vi "LIA Debugging FPGA.vi"() -> ()   [LabVIEW 2017]
uses:
  <instrlib>/_niInstr/Streaming/v1/Common/Stream State.ctl
  <instrlib>/_niInstr/Data Trigger/v1/Shared/Public/Edge Configuration FXP(+-,18,1).ctl
  <instrlib>/_niInstr/Data Trigger/v1/Shared/Public/Edge Configuration Trigger Slope.ctl
  LIA Decimator0 Enum.ctl
  LIA Decimator1 Enum.ctl
  Cascaded-SOS/FPGA/Controls/IIR_Coeffs.ctl
  <vilib>/Platform/TimedLoop/XDataNode/timing_clust.ctl
  <vilib>/Platform/TimedLoop/XDataNode/nitl_modes.ctl
  <vilib>/Platform/TimedLoop/XDataNode/wakeup.ctl
  <instrlib>/_niInstr/DSP/v1/Shared/Public/IQ Data.ctl
  <vilib>/rvi/Emulation/niFpgaSctlEmulationGetInTimedLoop.vi
  <vilib>/rvi/Emulation/niFpgaEmulationReportErrorSimple.vi
  <vilib>/rvi/Emulation/niFpgaGetClockAttributes.vi
  <vilib>/rvi/Emulation/niFpgaCriticalErrorInLSC.vi
  <instrlib>/_niInstr/DSP/v1/FPGA/Public/Sub VIs/Frequency Shift/Frequency Shift - 1 spc.vi
  <instrlib>/_niInstr/DSP/v1/FPGA/Public/Sub VIs/Fractional Decimator/Fractional Decimator - 1 spc - 2x oc.vi
  <instrlib>/_niInstr/DSP/v1/FPGA/Public/Sub VIs/Fractional Decimator/Fractional Decimator - 10 cps - 1x oc.vi
  <userlib>/_NI Noise Generation IP/FPGA/Public/Low Level/AWGN FXP23x2.vi
  <instrlib>/_niInstr/DSP/v1/FPGA/Public/Sub VIs/Frequency Shift/Frequency Shift - 2 spc.vi
  <vilib>/rvi/eio/common/nirviEmuTemplateMethod_errors.vi
  <vilib>/Platform/TimedLoop/XDataNode/XDataNode.xnode
  <instrlib>/_niInstr/DSP/v1/Xnodes/Public/Frequency Shift/niInstr DSP v1 Frequency Shift FPGA.xnode
  <vilib>/rvi/FXPMathLib/FxpMul/XNode/nifxpmath_Multiplier.xnode
  <vilib>/rvi/FXPMathLib/FxpAdd/XNode/nifxpmath_Add.xnode
  <vilib>/eio/EIONode/EIONode.xnode
  <vilib>/Platform/TimedLoop/XDataNode/XDNodeRunTimeDep.lvlib
  <instrlib>/_niInstr/Basic Elements/v1/FPGA/niInstr Basic Elements v1 FPGA.lvlib
  <instrlib>/_niInstr/DSP/v1/Shared/niInstr DSP v1 Shared.lvlib
  <instrlib>/_niInstr/DSP/v1/FPGA/niInstr DSP v1 FPGA.lvlib
  Program Files (x86)/National Instruments/LabVIEW 2017/examples/Lock-In Amplifier/_NI PLL IP/FPGA/NI PLL IP FPGA.lvlib
  Program Files (x86)/National Instruments/LabVIEW 2017/examples/Lock-In Amplifier/lib/fpga/Lock-In Amplifier Example FPGA.lvlib
  <instrlib>/_niInstr/Streaming/v1/Common/niInstr Streaming v1 Common.lvlib
  <userlib>/_NI Noise Generation IP/FPGA/NI Noise Generation IP FPGA v2.lvlib
  <vilib>/rvi/FXPMathLib/sim/FxpSim.dll
  <instrlib>/_niInstr/Data Trigger/v1/Shared/niInstr Data Trigger v1 Shared.lvlib
panel:
  in  "lock-in.iir enable0 0":bool
  in  "lock-in.iir enable1 0":bool
  in  "lock-in.iir config1 0":T1={"b0"=0.015777587890625, "b1"=-0.030517578125, "-a1"=1.9578399658203125, "-a2"=-0.9589080810546875}
  in  "lock-in.iir decimation1 0":fxp<+,4,4> format="%#_3g"
  in  "lock-in.iir decimation0 0":fxp<+,4,4> format="%#_3g"
  in  "lock-in.iir config0 0":T1={"b0"=0.015777587890625, "b1"=-0.030517578125, "-a1"=1.9578399658203125, "-a2"=-0.9589080810546875}
  in  "lock-in.decimator1 0":T2
  in  "lock-in.fir1 fs 0":fxp<+,48,1>
  in  "nco.enable 0":bool=TRUE
  in  "nco.reset 0":bool
  in  "nco.frequency 0":fxp<+/-,48,0>
  in  "lock-in.fir0 fs 0":fxp<+,48,1>
  in  "lock-in.decimator0 0":T3
  in  "dpll.reset 1":bool
  in  "dpll.enable 1":bool
  in  "dpll.q 1":fxp<+/-,48,0>
  in  "dpll.m 1":i8
  in  "dpll.config 1":T4
  out "dpll.vco output 1":fxp<+/-,48,0>
  in  "dpll.channel 1":i32
  in  "dpll.channel 0":i32
  out "dpll.vco output 0":fxp<+/-,48,0>
  in  "dpll.config 0":T4
  in  "dpll.m 0":i8
  in  "dpll.q 0":fxp<+/-,48,0>
  in  "dpll.enable 0":bool
  in  "dpll.reset 0":bool
  in  "lock-in.enable 3":bool
  in  "lock-in.enable 2":bool
  in  "lock-in.enable 1":bool
  in  "lock-in.carrier 3":fxp<+/-,48,0>
  in  "lock-in.carrier 2":fxp<+/-,48,0>
  in  "lock-in.enable 0":bool
  in  "lock-in.channel select 3":i32
  in  "lock-in.carrier select 3":i32
  in  "lock-in.cic config valid 3":bool
  in  "lock-in.cic config 3":cluster{"factor":fxp<+,16,16>, "shift":i16}
  in  "lock-in.reset 3":bool
  out "stream.state 3":T6 caption="stream.state 0"
  out "stream.samples transferred 3":u64 caption="stream.samples transferred 0"
  out "stream.metadata 3":u64 caption="stream.metadata 0"
  in  "stream.num samples 3":u64 caption="stream.num samples 0"
  in  "stream.request state 3":T6 caption="stream.request state 0"
  in  "lock-in.channel select 2":i32
  in  "lock-in.carrier select 2":i32
  in  "lock-in.cic config valid 2":bool
  in  "lock-in.cic config 2":cluster{"factor":fxp<+,16,16>, "shift":i16}
  in  "lock-in.reset 2":bool
  out "stream.state 2":T6 caption="stream.state 0"
  out "stream.samples transferred 2":u64 caption="stream.samples transferred 0"
  out "stream.metadata 2":u64 caption="stream.metadata 0"
  in  "stream.num samples 2":u64 caption="stream.num samples 0"
  in  "stream.request state 2":T6 caption="stream.request state 0"
  out "pll.vco output 0":fxp<+/-,48,0>
  out "pll.vco output 1":fxp<+/-,48,0>
  out "stream.metadata 4":u64 caption="stream.metadata 0"
  out "stream.samples transferred 4":u64 caption="stream.samples transferred 0"
  out "stream.state 4":T6 caption="stream.state 0"
  in  "stream.request state 4":T6 caption="stream.request state 0"
  in  "stream.num samples 4":u64 caption="stream.num samples 0"
  in  "preview.channel select":i32
  in  "ao.reset 3":bool
  in  "ao.carrier 2":fxp<+/-,48,0>=0.010000000000001563
  in  "ao.level 2":fxp<+/-,18,1>
  in  "ao.reset 2":bool
  in  "ao.carrier 1":fxp<+/-,48,0>=0.010000000000001563
  in  "ao.level 1":fxp<+/-,18,1>
  in  "ao.reset 1":bool
  in  "ao.reset 0":bool
  in  "ao.carrier 0":fxp<+/-,48,0>=0.010000000000001563
  in  "ao.level 0":fxp<+/-,18,1>
  in  "lock-in.channel select 1":i32
  in  "lock-in.channel select 0":i32
  in  "stream.request state 1":T6 caption="stream.request state 0"
  in  "stream.num samples 1":u64 caption="stream.num samples 0"
  out "stream.metadata 1":u64 caption="stream.metadata 0"
  out "stream.samples transferred 1":u64 caption="stream.samples transferred 0"
  out "stream.state 1":T6 caption="stream.state 0"
  in  "lock-in.reset 1":bool
  in  "lock-in.cic config 1":cluster{"factor":fxp<+,16,16>, "shift":i16}
  in  "lock-in.cic config valid 1":bool
  in  "lock-in.carrier select 1":i32
  in  "lock-in.carrier select 0":i32
  in  "lock-in.cic config valid 0":bool
  in  "lock-in.cic config 0":cluster{"factor":fxp<+,16,16>, "shift":i16}
  in  "lock-in.reset 0":bool
  in  "lock-in.carrier 1":fxp<+/-,48,0>
  in  "lock-in.carrier 0":fxp<+/-,48,0>
  in  "ao.level 3":fxp<+/-,18,1>
  in  "pll.channel 1":i32
  in  "pll.reset 1":bool
  in  "pll.enable 1":bool
  in  "pll.config 1":T7={"quiescent frequency"=0.10000000000000142, "compensation"=0.0, "psd gain"=-18, "loop filter"={"order"=4, "cutoff"=6}}
  in  "pll.channel 0":i32
  in  "ao.noise gain 3":fxp<+,18,1>=0.01000213623046875
  in  "ao.carrier 3":fxp<+/-,48,0>=0.010000000000001563
  in  "ao.noise seeds 3":fxp<+,23,23>[](array[numeric])=[1.0, 12323.0]
  in  "pll.reset 0":bool
  in  "pll.enable 0":bool
  in  "stream.request state 0":T6
  in  "stream.num samples 0":u64
  out "stream.metadata 0":u64
  out "stream.samples transferred 0":u64
  out "stream.state 0":T6
  in  "pll.config 0":T7={"quiescent frequency"=0.10000000000000142, "compensation"=0.0, "psd gain"=-18, "loop filter"={"order"=4, "cutoff"=6}}
  out "IO Module\\InitDone":bool
  out "IO Module\\User Error":u32
  in  "IO Module\\User Command":u32
  in  "IO Module\\User Command Valid":bool
  out "IO Module\\User Command Ready":bool
  in  "IO Module\\User Command Arg 0":u32
  in  "IO Module\\User Command Arg 1":u32
  out "IO Module\\User Command Error":u16
  out "IO Module\\User Command Return":u32
  out "IO Module\\User Command Return Valid":bool
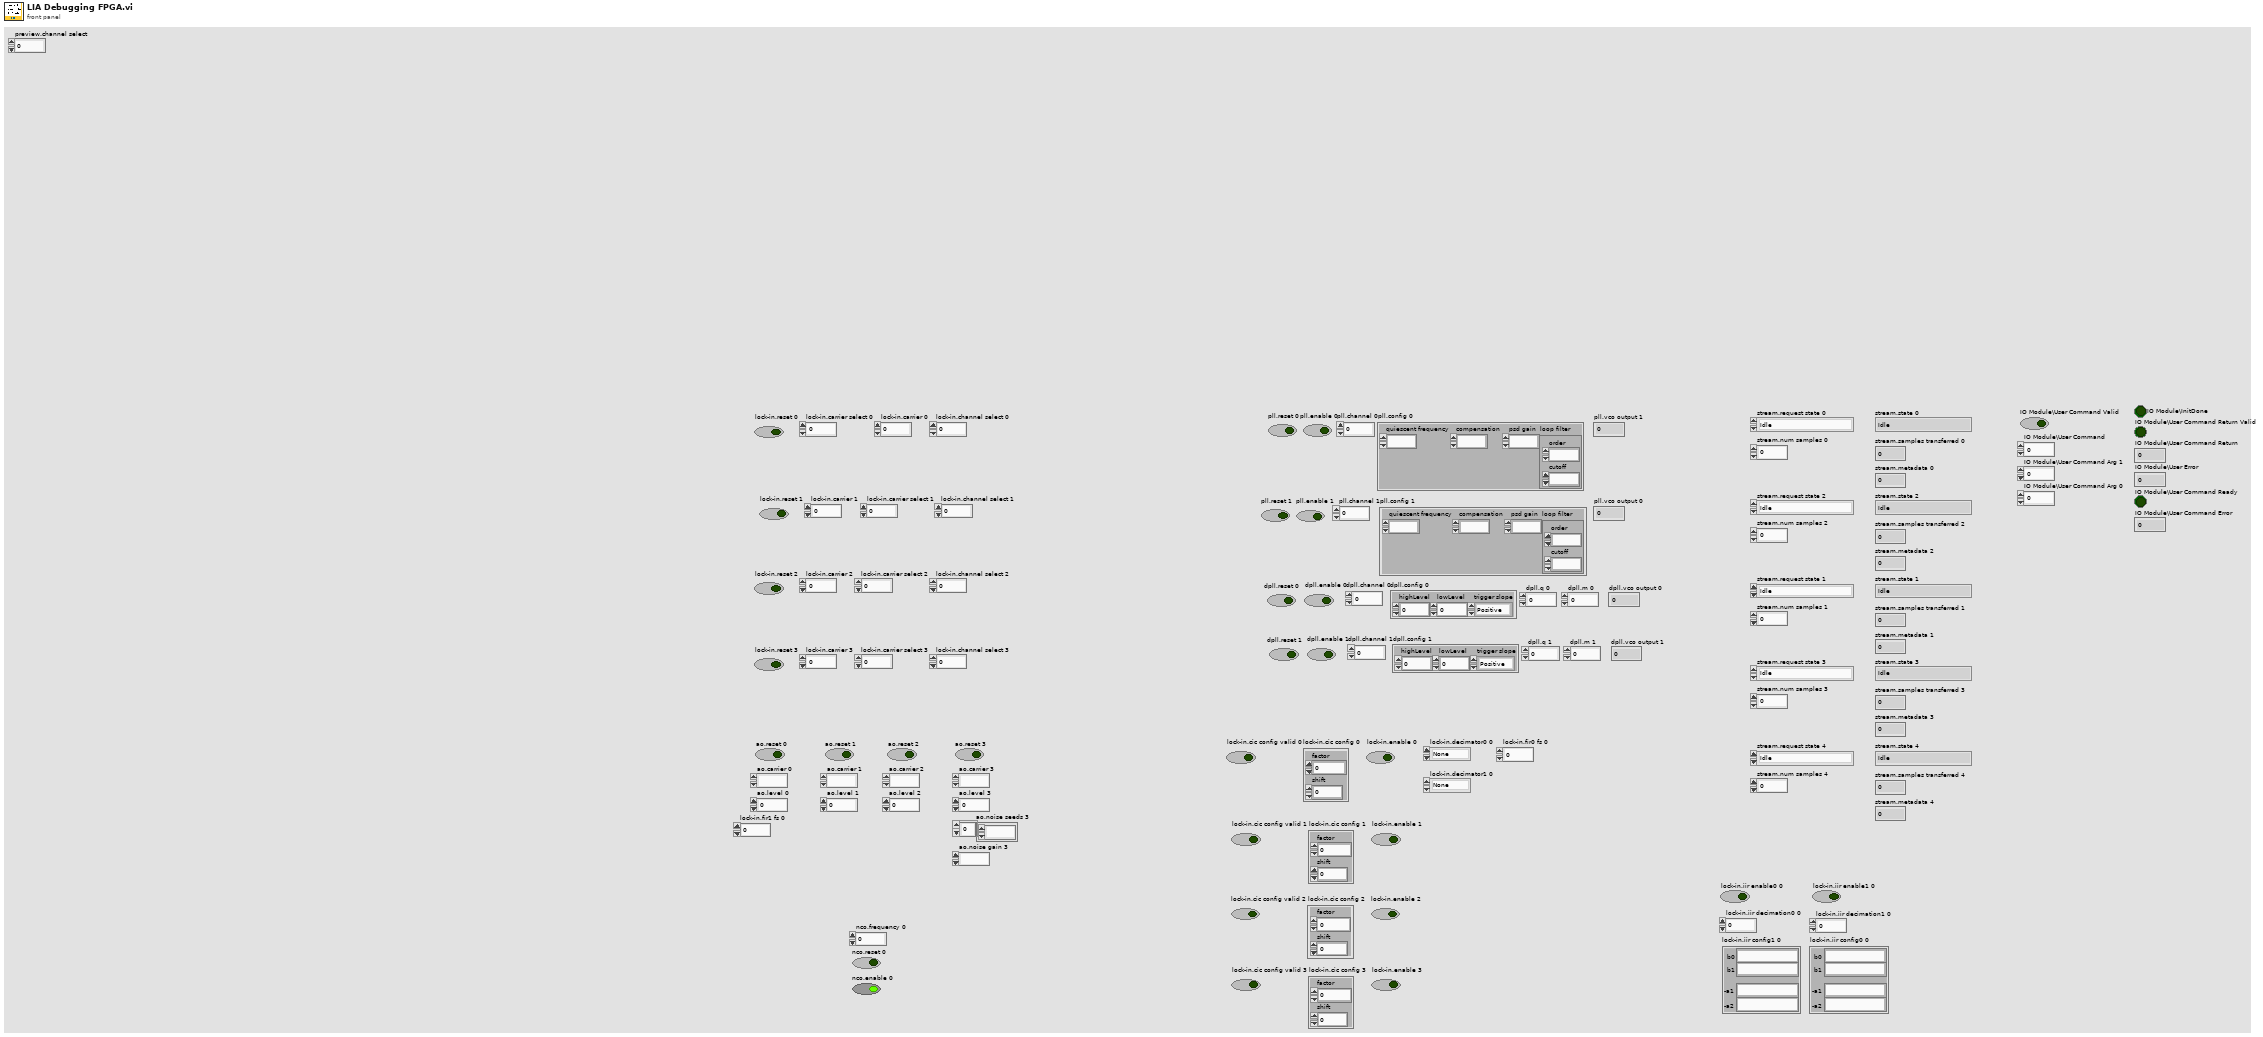
[diagram p1: front panel]
types:
  T1 = typedef "IIR_Coeffs.ctl" = cluster{"b0":fxp<+/-,18,2>, "b1":fxp<+/-,18,2>, "-a1":fxp<+/-,18,2>, "-a2":fxp<+/-,18,2>}
  T2 = typedef "LIA Decimator1 Enum.ctl" = enum16{"None", "FIR", "SOS"}
  T3 = typedef "LIA Decimator0 Enum.ctl" = enum16{"None", "CIC", "FIR", "4HB", "SOS"}
  T4 = typedef "niInstr Data Trigger v1 Shared.lvlib/Edge Configuration FXP(+-,18,1).ctl" = cluster{"highLevel":fxp<+/-,18,1>, "lowLevel":fxp<+/-,18,1>, "trigger slope":T5}
  T5 = typedef "niInstr Data Trigger v1 Shared.lvlib/Edge Configuration Trigger Slope.ctl" = enum8{"Positive", "Negative"}
  T6 = typedef "niInstr Streaming v1 Common.lvlib/Stream State.ctl" = enum8{"Idle", "Finite Transfer", "Continuous", "Done", "Error", "Not Ready", "Cancel"}
  T7 = cluster{"quiescent frequency":fxp<+/-,48,0>, "compensation":fxp<+/-,18,3>, "psd gain":i16, "loop filter":cluster{"order":i32, "cutoff":i8}}
  T8 = typedef "XDNodeRunTimeDep.lvlib/timing_clust.ctl" = cluster{"Expected End [f-1]":u64, "Actual End [f-1]":u64, "Finished Late? [f-1]":bool, "Expected End [i-1]":u64, "Actual End [i-1]":u64, "Finished Late? [i-1]":bool, "Expected Start [i]":u64, "Actual Start [i]":u64, "Expected Start [f]":u64, "Actual Start [f]":u64, "Source Name":string, "Structure Name":string, "Period":i64, "Deadline":i64, "Offset":i64, "Start":i64, "Priority":i32, "Timeout":i32, "Mode":T9, "Wakeup Reason":T10, "Error":errorcluster, "Source Type":string, "Secondary Source Type":string, "Global End Time":u64, "Global Start Time":u64, "Frame Duration":u64, "Iteration Duration":u64, "Assigned CPU":i32, "I/O Scan Engine Mode":u32}
  T9 = typedef "XDNodeRunTimeDep.lvlib/nitl_modes.ctl" = enum32{"No Change", "Process missed periods, maintain original phase", "Discard missed periods, maintain original phase", "Process missed periods, ignore original phase", "Discard missed periods, ignore original phase"}
  T10 = typedef "XDNodeRunTimeDep.lvlib/wakeup.ctl" = enum32{"Normal", "Aborted", "Asynchronous wakeup", "Timing source error", "Timed loop error", "Timeout"}
  T11 = cluster{"stream.num samples 0":u64, "stream.request state 0":T6, "stream.index 0":i16}
  T12 = typedef "niInstr DSP v1 Shared.lvlib/IQ Data.ctl" = cluster{"I":fxp<+/-,18,1>, "Q":fxp<+/-,18,1>, "overflow":bool}
  T13 = cluster{"stream.metadata 0":u64, "stream.samples transferred 0":u64, "stream.state 0":T6}
  T14 = typedef "niInstr DSP v1 Shared.lvlib/IQ Data - 25 bit.ctl" = cluster{"I":fxp<+/-,25,1>, "Q":fxp<+/-,25,1>, "overflow":bool}
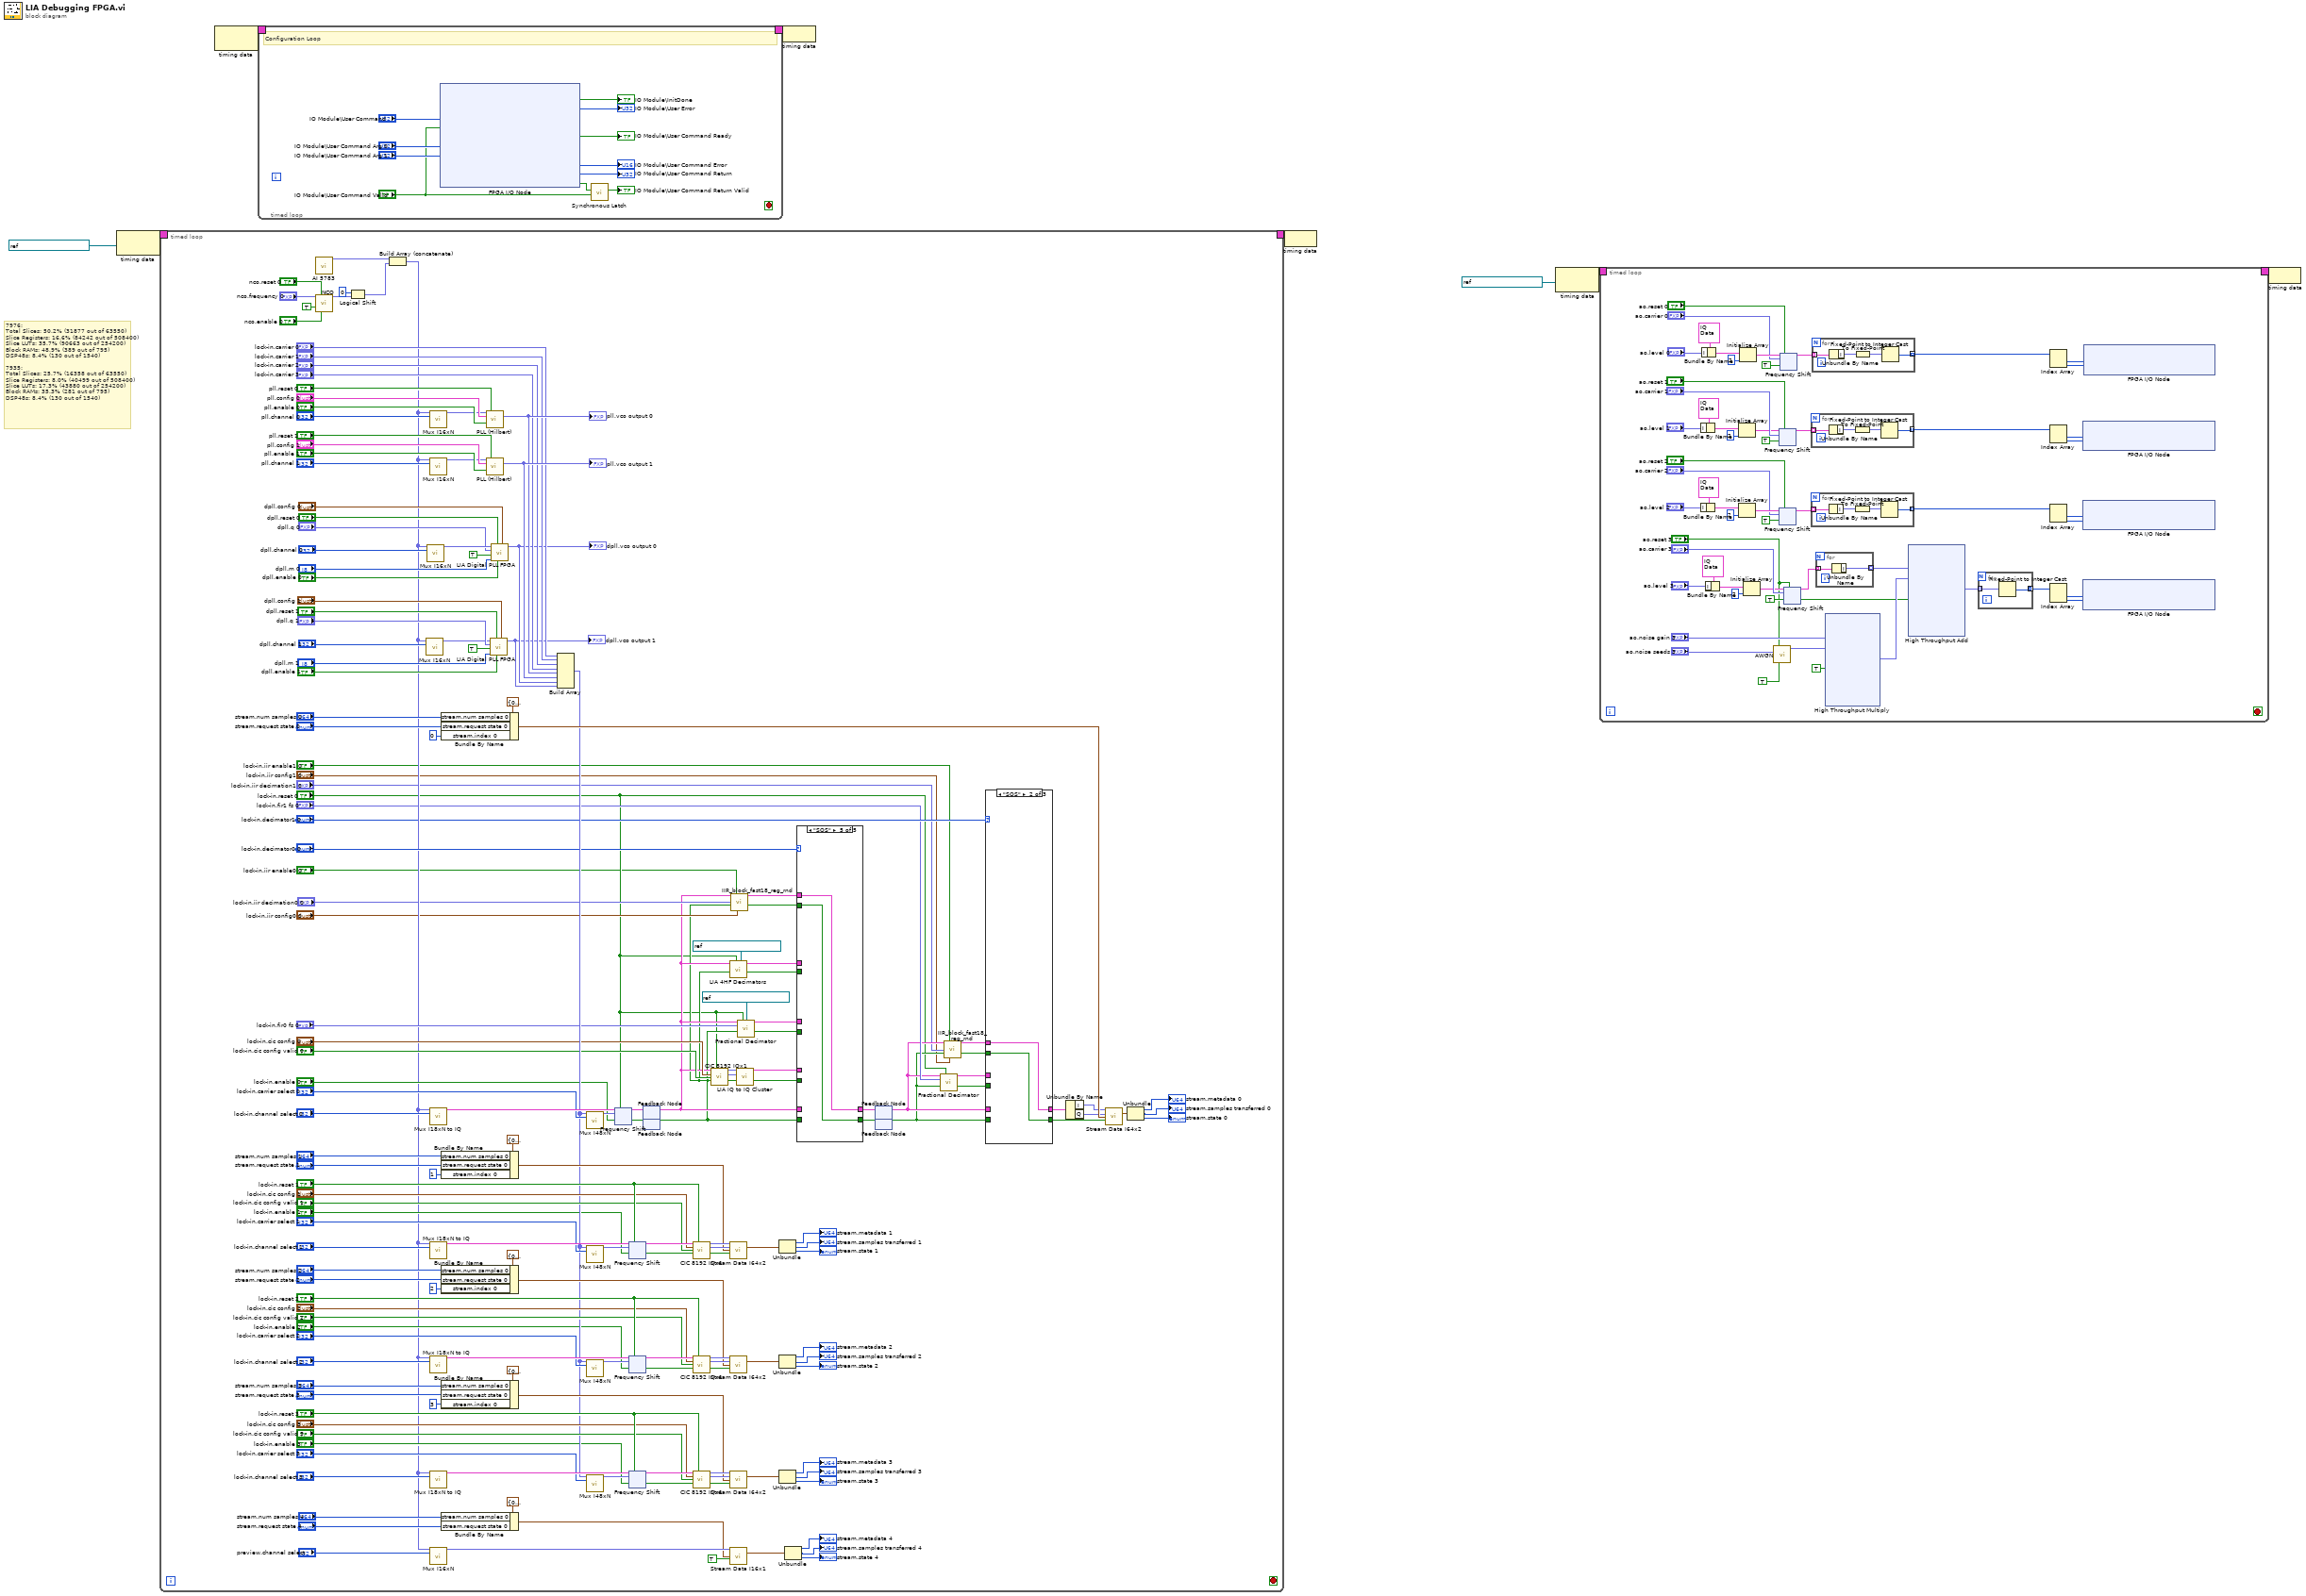
[diagram p0: block diagram]
diagram:
  # "7976:\nTotal Slices: 50.2% (31877 out of 63550)\nSlice Registers: 16.6% (84242 out of 508400)\nSlice LUTs: 35.7% (90663 out of 254200)\nBlock RAMs: 48.9% (389 out of 795)\nDSP48s: 8.4% (130 out of 1540)\n\n7935:\nTotal Slices: 25.7% (16358 out of 63550)\nSlice Registers: 8.0% (40499 out of 508400)\nSlice LUTs: 17.3% (43880 out of 254200)\nBlock RAMs: 35.3% (281 out of 795)\nDSP48s: 8.4% (130 out of 1540)"
  n1 = node-c288(refnum<k21> "IO Module\\Data Clock" ("Source Name")) -> (w8:T8)
  n2 = timed-loop {
    timing: w8 -> [_]
    timing-out: [_] -> w7
    stop <- _ stop-if-true
    n3 = call "AI 5783.vi"() -> ("i18x1"=w59:fxp<+/-,18,1>[])  [unwired: 14 in, 1 out]
    n4 = call <instrlib>:"NCO.vi"("frequency"="nco.frequency 0", "reset"="nco.reset 0", "input valid"=TRUE, "enable (T)"="nco.enable 0") -> ("cosine out"=w29:fxp<+/-,18,1>)  [unwired: 9 in, 2 out]
    n5 = Logical Shift(y=i16 0, x=w29) -> (x << y=w30:fxp<+/-,18,1>)
    n6 = Build Array (concatenate)(w59, w30) -> (w52:fxp<+/-,18,1>[])
    n7 = call "Mux I16xN.vi"("i16xn in"=w52, "index"="dpll.channel 1") -> ("i16 out"=w62:fxp<+/-,18,1>)  [unwired: 12 in, 1 out]
    n8 = call "Mux I16xN.vi"("i16xn in"=w52, "index"="dpll.channel 0") -> ("i16 out"=w74:fxp<+/-,18,1>)  [unwired: 12 in, 1 out]
    n9 = call "Mux I16xN.vi"("i16xn in"=w52, "index"="pll.channel 0") -> ("i16 out"=w181:fxp<+/-,18,1>)  [unwired: 12 in, 1 out]
    n10 = call "Mux I16xN.vi"("i16xn in"=w52, "index"="pll.channel 1") -> ("i16 out"=w175:fxp<+/-,18,1>)  [unwired: 12 in, 1 out]
    n11 = call "Mux I18xN to IQ.vi"("i16xn in"=w52, "index"="lock-in.channel select 0") -> ("output"=w174:T12)  [unwired: 12 in, 1 out]
    n12 = call "Mux I18xN to IQ.vi"("i16xn in"=w52, "index"="lock-in.channel select 1") -> ("output"=w161:T12)  [unwired: 12 in, 1 out]
    n13 = call "Mux I18xN to IQ.vi"("i16xn in"=w52, "index"="lock-in.channel select 2") -> ("output"=w127:T12)  [unwired: 12 in, 1 out]
    n14 = call "Mux I18xN to IQ.vi"("i16xn in"=w52, "index"="lock-in.channel select 3") -> ("output"=w106:T12)  [unwired: 12 in, 1 out]
    n15 = call "Mux I16xN.vi"("i16xn in"=w52, "index"="preview.channel select") -> ("i16 out"=w135:fxp<+/-,18,1>)  [unwired: 12 in, 1 out]
    n16 = Bundle By Name(cluster=T11 {"stream.num samples 0"=0, "stream.request state 0"=enum."Idle", "stream.index 0"=0} ("config"), "stream.num samples 0"="stream.num samples 0", "stream.request state 0"="stream.request state 0", "stream.index 0"=i16 0) -> (w164:T11)
    n17 = Bundle By Name(cluster=T11 {"stream.num samples 0"=0, "stream.request state 0"=enum."Idle", "stream.index 0"=0} ("config"), "stream.num samples 0"="stream.num samples 1", "stream.request state 0"="stream.request state 1", "stream.index 0"=i16 1) -> (w143:T11)
    n18 = Bundle By Name(cluster=T11 {"stream.num samples 0"=0, "stream.request state 0"=enum."Idle", "stream.index 0"=0} ("config"), "stream.num samples 0"="stream.num samples 2", "stream.request state 0"="stream.request state 2", "stream.index 0"=i16 2) -> (w109:T11)
    n19 = Bundle By Name(cluster=T11 {"stream.num samples 0"=0, "stream.request state 0"=enum."Idle", "stream.index 0"=0} ("config"), "stream.num samples 0"="stream.num samples 3", "stream.request state 0"="stream.request state 3", "stream.index 0"=i16 3) -> (w88:T11)
    n20 = Bundle By Name(cluster=T11 {"stream.num samples 0"=0, "stream.request state 0"=enum."Idle", "stream.index 0"=0} ("config"), "stream.num samples 0"="stream.num samples 4", "stream.request state 0"="stream.request state 4") -> (w131:T11)
    n21 = call "PLL (Hilbert).vi"("input"=w181, "reset"="pll.reset 0", "config"="pll.config 0", "enable"="pll.enable 0") -> ("output"=w128:fxp<+/-,48,0>)  [unwired: 11 in]
    "pll.vco output 0" <- w128
    n22 = call "PLL (Hilbert).vi"("input"=w175, "reset"="pll.reset 1", "config"="pll.config 1", "enable"="pll.enable 1") -> ("output"=w129:fxp<+/-,48,0>)  [unwired: 11 in]
    "pll.vco output 1" <- w129
    n23 = call "LIA Digital PLL FPGA.vi"("configuration"="dpll.config 1", "arm"="dpll.enable 1", "reset"="dpll.reset 1", "m"="dpll.m 1", "input valid"=TRUE, "q"="dpll.q 1", "I"=w62) -> ("frequency shift"=w58:fxp<+/-,48,0>)  [unwired: 1 in, 3 out]
    "dpll.vco output 1" <- w58
    n24 = call "LIA Digital PLL FPGA.vi"("configuration"="dpll.config 0", "arm"="dpll.enable 0", "reset"="dpll.reset 0", "m"="dpll.m 0", "input valid"=TRUE, "q"="dpll.q 0", "I"=w74) -> ("frequency shift"=w69:fxp<+/-,48,0>)  [unwired: 1 in, 3 out]
    "dpll.vco output 0" <- w69
    n25 = Build Array("lock-in.carrier 0", "lock-in.carrier 1", "lock-in.carrier 2", "lock-in.carrier 3", w128, w129, w69, w58) -> (w85:fxp<+/-,48,0>[])
    n26 = call "Mux I48xN.vi"("i48xn in"=w85, "index"="lock-in.carrier select 0") -> ("i48 out"=w173:fxp<+/-,48,0>)  [unwired: 13 in]
    n27 = call "Mux I48xN.vi"("i48xn in"=w85, "index"="lock-in.carrier select 1") -> ("i48 out"=w160:fxp<+/-,48,0>)  [unwired: 13 in]
    n28 = call "Mux I48xN.vi"("i48xn in"=w85, "index"="lock-in.carrier select 2") -> ("i48 out"=w126:fxp<+/-,48,0>)  [unwired: 13 in]
    n29 = call "Mux I48xN.vi"("i48xn in"=w85, "index"="lock-in.carrier select 3") -> ("i48 out"=w105:fxp<+/-,48,0>)  [unwired: 13 in]
    n30 = xnode "Frequency Shift"("data in"=w174, "reset"="lock-in.reset 0", "frequency shift"=w173, "input valid"="lock-in.enable 0") -> ("data out"=w27:T12, "output valid"=w25:bool)  [unwired: 2 in, 1 out]
    n31 = xnode "Frequency Shift"("data in"=w161, "reset"="lock-in.reset 1", "frequency shift"=w160, "input valid"="lock-in.enable 1") -> ("data out"=w159:T12, "output valid"=w158:bool)  [unwired: 2 in, 1 out]
    n32 = xnode "Frequency Shift"("data in"=w127, "reset"="lock-in.reset 2", "frequency shift"=w126, "input valid"="lock-in.enable 2") -> ("data out"=w125:T12, "output valid"=w124:bool)  [unwired: 2 in, 1 out]
    n33 = xnode "Frequency Shift"("data in"=w106, "reset"="lock-in.reset 3", "frequency shift"=w105, "input valid"="lock-in.enable 3") -> ("data out"=w104:T12, "output valid"=w103:bool)  [unwired: 2 in, 1 out]
    n34 = feedback-in #1(w27) -> ()
    n35 = feedback #1() -> (w19:T12)  [unwired: 1 in]
    n36 = feedback-in #2(w25) -> ()
    n37 = feedback #2() -> (w18:bool)  [unwired: 1 in]
    n38 = call "CIC 8192 IQx1.vi"("data"=w159, "reset"="lock-in.reset 1", "config"="lock-in.cic config 1", "config valid"="lock-in.cic config valid 1", "input valid"=w158) -> ("i out"=w154:fxp<+/-,64,1>, "q out"=w153:fxp<+/-,64,1>, "output valid"=w152:bool)  [unwired: 8 in]
    n39 = call "CIC 8192 IQx1.vi"("data"=w125, "reset"="lock-in.reset 2", "config"="lock-in.cic config 2", "config valid"="lock-in.cic config valid 2", "input valid"=w124) -> ("i out"=w120:fxp<+/-,64,1>, "q out"=w119:fxp<+/-,64,1>, "output valid"=w118:bool)  [unwired: 8 in]
    n40 = call "CIC 8192 IQx1.vi"("data"=w104, "reset"="lock-in.reset 3", "config"="lock-in.cic config 3", "config valid"="lock-in.cic config valid 3", "input valid"=w103) -> ("i out"=w99:fxp<+/-,64,1>, "q out"=w98:fxp<+/-,64,1>, "output valid"=w97:bool)  [unwired: 8 in]
    n41 = call "CIC 8192 IQx1.vi"("data"=w19, "reset"="lock-in.reset 0", "config"="lock-in.cic config 0", "config valid"="lock-in.cic config valid 0", "input valid"=w18) -> ("i out"=w36:fxp<+/-,64,1>, "q out"=w35:fxp<+/-,64,1>, "output valid"=w54:bool)  [unwired: 8 in]
    n42 = call "LIA 4HF Decimators.vi"("clock x 2"=refnum<k21> "IO Module\\Data Clock 2x", "reset"="lock-in.reset 0", "input valid"=w18, "data in"=w19) -> ("output valid"=w43:bool, "data out"=w44:T12)  [unwired: 6 in]
    n43 = call "Stream Data I64x2.vi"("i in"=w154, "q in"=w153, "config"=w143, "input valid"=w152) -> ("status"=w151:T13)  [unwired: 11 in]
    n44 = call "Stream Data I64x2.vi"("i in"=w120, "q in"=w119, "config"=w109, "input valid"=w118) -> ("status"=w117:T13)  [unwired: 11 in]
    n45 = call "Stream Data I64x2.vi"("i in"=w99, "q in"=w98, "config"=w88, "input valid"=w97) -> ("status"=w96:T13)  [unwired: 11 in]
    n46 = call "Stream Data I16x1.vi"("i in"=w135, "config"=w131, "input valid"=TRUE) -> ("status"=w137:T13)  [unwired: 12 in]
    n47 = call "IIR_block_fast18_reg_rnd.vi"("IQ_Data_In"=w19, "enable"="lock-in.iir enable0 0", "Decimation Factor (-1)"="lock-in.iir decimation0 0", "Valid In"=w18, "IIR 2 coeffs"="lock-in.iir config0 0") -> ("IQ_Data_Out"=w26:T12, "output valid"=w24:bool)  [unwired: 9 in]
    n48 = call "LIA IQ to IQ Cluster.vi"("i in"=w36, "q in"=w35) -> ("data out"=w34:T12)  [unwired: 13 in]
    n49 = call-poly <instrlib>:"Fractional Decimator.vi"("data in"=w19, "reset"="lock-in.reset 0", "clock x 2"=refnum<k21> "IO Module\\Data Clock 2x", "output sample rate"="lock-in.fir0 fs 0", "input valid"=w18) -> ("data out"=w46:T12, "output valid"=w47:bool)  [unwired: 8 in, 1 out]
    n50 = Unbundle(w151) -> ("stream.metadata 0"=→"stream.metadata 1":u64, "stream.samples transferred 0"=→"stream.samples transferred 1":u64, "stream.state 0"=→"stream.state 1":T6)
    n51 = Unbundle(w117) -> ("stream.metadata 0"=→"stream.metadata 2":u64, "stream.samples transferred 0"=→"stream.samples transferred 2":u64, "stream.state 0"=→"stream.state 2":T6)
    n52 = Unbundle(w96) -> ("stream.metadata 0"=→"stream.metadata 3":u64, "stream.samples transferred 0"=→"stream.samples transferred 3":u64, "stream.state 0"=→"stream.state 3":T6)
    n53 = Unbundle(w137) -> ("stream.metadata 0"=→"stream.metadata 4":u64, "stream.samples transferred 0"=→"stream.samples transferred 4":u64, "stream.state 0"=→"stream.state 4":T6)
    n54 = case shown="\"SOS\"" "lock-in.decimator0 0" {
      tunnel: [w192 w194 w196 w198 w199] -> w15
      tunnel: w54 -> [_ w194 _ _ _]
      tunnel: w47 -> [_ _ w196 _ _]
      tunnel: w18 -> [w192 _ _ _ _]
      tunnel: w46 -> [_ _ w195 _ _]
      tunnel: w19 -> [w191 _ _ _ _]
      tunnel: w44 -> [_ _ _ w197 _]
      tunnel: w43 -> [_ _ _ w198 _]
      tunnel: [w191 w193 w195 w197 w200] -> w17
      tunnel: w34 -> [_ w193 _ _ _]
      tunnel: w26 -> [_ _ _ _ w200]
      tunnel: w24 -> [_ _ _ _ w199]
      frame "None", Default {
      }
      frame "CIC" {
      }
      frame "FIR" {
      }
      frame "4HB" {
      }
      frame "SOS" {
      }
    }
    n55 = feedback #3() -> (w16:T12)  [unwired: 1 in]
    n56 = feedback-in #3(w17) -> ()
    n57 = feedback #4() -> (w14:bool)  [unwired: 1 in]
    n58 = feedback-in #4(w15) -> ()
    n59 = call-poly <instrlib>:"Fractional Decimator.vi"("data in"=w16, "reset"="lock-in.reset 0", "output sample rate"="lock-in.fir1 fs 0", "input valid"=w14) -> ("data out"=w33:T14, "output valid"=w32:bool)  [unwired: 9 in, 1 out]
    n60 = call "IIR_block_fast18_reg_rnd.vi"("IQ_Data_In"=w16, "enable"="lock-in.iir enable1 0", "Decimation Factor (-1)"="lock-in.iir decimation1 0", "Valid In"=w14, "IIR 2 coeffs"="lock-in.iir config1 0") -> ("IQ_Data_Out"=w23:T12, "output valid"=w22:bool)  [unwired: 9 in]
    n61 = case shown="\"SOS\"" "lock-in.decimator1 0" {
      tunnel: [w185 w187 w190] -> w42
      tunnel: w14 -> [_ _ w190]
      tunnel: w16 -> [_ _ w189]
      tunnel: [w186 w188 w189] -> w40
      tunnel: w33 -> [w186 _ _]
      tunnel: w32 -> [w185 _ _]
      tunnel: w23 -> [_ w188 _]
      tunnel: w22 -> [_ w187 _]
      frame "FIR" {
      }
      frame "SOS" {
      }
      frame "None", Default {
      }
    }
    n62 = Unbundle By Name(w40) -> ("I"=w39:fxp<+/-,25,1>, "Q"=w38:fxp<+/-,25,1>)
    n63 = call "Stream Data I64x2.vi"("i in"=w39, "q in"=w38, "config"=w164, "input valid"=w42) -> ("status"=w172:T13)  [unwired: 11 in]
    n64 = Unbundle(w172) -> ("stream.metadata 0"=→"stream.metadata 0":u64, "stream.samples transferred 0"=→"stream.samples transferred 0":u64, "stream.state 0"=→"stream.state 0":T6)
  }
  n65 = node-c288() -> (w2:T8)  [unwired: 1 in]
  n66 = timed-loop {
    timing: w2 -> [_]
    timing-out: [_] -> w1
    stop <- _ stop-if-true
    # "Configuration Loop"
    n67 = xnode "FPGA I/O Node"("IO Module\\User Command"="IO Module\\User Command", "IO Module\\User Command Valid"="IO Module\\User Command Valid", "IO Module\\User Command Arg 0"="IO Module\\User Command Arg 0", "IO Module\\User Command Arg 1"="IO Module\\User Command Arg 1") -> ("IO Module\\InitDone"=→"IO Module\\InitDone":bool, "IO Module\\Clip Error Code"=→"IO Module\\User Error":u32, "IO Module\\User Command Ready"=→"IO Module\\User Command Ready":bool, "IO Module\\User Command Error"=→"IO Module\\User Command Error":u16, "IO Module\\User Command Return"=→"IO Module\\User Command Return":u32, "IO Module\\User Command Return Valid"=w240:bool)  [unwired: 10 in, 10 out]
    n68 = call <instrlib>:"Synchronous Latch.vi"("clear"="IO Module\\User Command Valid", "set"=w240) -> ("out"=→"IO Module\\User Command Return Valid":bool)  [unwired: 9 in]
  }
  n69 = node-c288(w1) -> ()
  n70 = node-c288(w7) -> ()
  n71 = node-c288(refnum<k21> "IO Module\\Data Clock" ("Source Name")) -> (w5:T8)
  n72 = timed-loop {
    timing: w5 -> [_]
    timing-out: [_] -> w4
    stop <- _ stop-if-true
    n73 = Bundle By Name(cluster=T12 {"I"=0.0, "Q"=0.0, "overflow"=FALSE} ("output"), "I"="ao.level 1") -> (w273:T12)
    n74 = Bundle By Name(cluster=T12 {"I"=0.0, "Q"=0.0, "overflow"=FALSE} ("output"), "I"="ao.level 2") -> (w263:T12)
    n75 = Bundle By Name(cluster=T12 {"I"=0.0, "Q"=0.0, "overflow"=FALSE} ("output"), "I"="ao.level 0") -> (w288:T12)
    n76 = Bundle By Name(cluster=T12 {"I"=0.0, "Q"=0.0, "overflow"=FALSE} ("output"), "I"="ao.level 3") -> (w297:T12)
    n77 = Initialize Array(w273, 2 ("dimension size")) -> (w269:T12[])
    n78 = Initialize Array(w263, 2 ("dimension size")) -> (w267:T12[])
    n79 = Initialize Array(w288, 2 ("dimension size")) -> (w292:T12[])
    n80 = Initialize Array(w297, 2 ("dimension size")) -> (w293:T12[])
    n81 = call-poly <userlib>:"AWGN.vi"("reset"="ao.reset 3", "seeds"="ao.noise seeds 3", "ready"=TRUE) -> ("output 0"=w300:fxp<+/-,23,4>[])  [unwired: 10 in, 2 out]
    n82 = xnode "Frequency Shift"("data in"=w269, "reset"="ao.reset 1", "frequency shift"="ao.carrier 1", "input valid"=TRUE) -> ("data out"=w277:T12[])  [unwired: 2 in, 2 out]
    n83 = xnode "Frequency Shift"("data in"=w267, "reset"="ao.reset 2", "frequency shift"="ao.carrier 2", "input valid"=TRUE) -> ("data out"=w259:T12[])  [unwired: 2 in, 2 out]
    n84 = xnode "Frequency Shift"("data in"=w292, "reset"="ao.reset 0", "frequency shift"="ao.carrier 0", "input valid"=TRUE) -> ("data out"=w284:T12[])  [unwired: 2 in, 2 out]
    n85 = xnode "Frequency Shift"("data in"=w293, "reset"="ao.reset 3", "frequency shift"="ao.carrier 3", "input valid"=TRUE) -> ("data out"=w308:T12[], "output valid"=w305:bool)  [unwired: 2 in, 1 out]
    n86 = for {
      tunnel: w277 -> [w324] mode=indexing
      tunnel: [w325] -> w278 mode=indexing
      n87 = Unbundle By Name(w324) -> ("I"=w323:fxp<+/-,18,1>)
      n88 = To Fixed-Point(number=w323) -> (fixed-point=w322:fxp<+/-,16,1>)  [unwired: 1 in]
      n89 = Fixed-Point to Integer Cast(1:w322) -> (0:w325:i16)
    }
    n90 = for {
      tunnel: w259 -> [w311] mode=indexing
      tunnel: [w312] -> w258 mode=indexing
      n91 = Unbundle By Name(w311) -> ("I"=w310:fxp<+/-,18,1>)
      n92 = To Fixed-Point(number=w310) -> (fixed-point=w309:fxp<+/-,16,1>)  [unwired: 1 in]
      n93 = Fixed-Point to Integer Cast(1:w309) -> (0:w312:i16)
    }
    n94 = for {
      tunnel: w284 -> [w337] mode=indexing
      tunnel: [w338] -> w283 mode=indexing
      n95 = Unbundle By Name(w337) -> ("I"=w336:fxp<+/-,18,1>)
      n96 = To Fixed-Point(number=w336) -> (fixed-point=w335:fxp<+/-,16,1>)  [unwired: 1 in]
      n97 = Fixed-Point to Integer Cast(1:w335) -> (0:w338:i16)
    }
    n98 = for {
      tunnel: w308 -> [w351] mode=indexing
      tunnel: [w350] -> w304 mode=indexing
      n99 = Unbundle By Name(w351) -> ("I"=w350:fxp<+/-,18,1>)
    }
    n100 = xnode ("High Throughput Multiply")("x"="ao.noise gain 3", "y"=w300, "input valid"=TRUE) -> ("x*y"=w307:fxp<+/-,41,5>[])  [unwired: 1 in, 2 out]
    n101 = xnode ("High Throughput Add")("x"=w304, "y"=w307, "input valid"=w305) -> ("x+y"=w299:fxp<+/-,16,1>[])  [unwired: 1 in, 2 out]
    n102 = for {
      tunnel: w299 -> [w349] mode=indexing
      tunnel: [w348] -> w268 mode=indexing
      n103 = Fixed-Point to Integer Cast(1:w349) -> (0:w348:i16)
    }
    n104 = Index Array(array=w283) -> (element #1=w282:i16, element #2=w281:i16)  [unwired: 2 in]
    n105 = Index Array(array=w278) -> (element #1=w279:i16, element #2=w280:i16)  [unwired: 2 in]
    n106 = Index Array(array=w258) -> (element #1=w257:i16, element #2=w256:i16)  [unwired: 2 in]
    n107 = Index Array(array=w268) -> (element #1=w255:i16, element #2=w254:i16)  [unwired: 2 in]
    n108 = xnode "FPGA I/O Node"("IO Module\\AO 1 Data N-1 Data Clock"=w279, "IO Module\\AO 1 Data N Data Clock"=w280) -> ()  [unwired: 2 in, 2 out]
    n109 = xnode "FPGA I/O Node"("IO Module\\AO 2 Data N-1 Data Clock"=w257, "IO Module\\AO 2 Data N Data Clock"=w256) -> ()  [unwired: 2 in, 2 out]
    n110 = xnode "FPGA I/O Node"("IO Module\\AO 3 Data N-1 Data Clock"=w255, "IO Module\\AO 3 Data N Data Clock"=w254) -> ()  [unwired: 2 in, 2 out]
    n111 = xnode "FPGA I/O Node"("IO Module\\AO 0 Data N-1 Data Clock"=w282, "IO Module\\AO 0 Data N Data Clock"=w281) -> ()  [unwired: 2 in, 2 out]
  }
  n112 = node-c288(w4) -> ()
